vi "IndependentVISApowerDataCollection.vi"() -> ()   [LabVIEW 2019]
uses:
  <vilib>/Utility/file.llb/Write Delimited Spreadsheet (string).vi
  <vilib>/Utility/file.llb/Read Delimited Spreadsheet (string).vi
  <instrlib>/niDigital/niDigital.llb/niDigital Selected Function.ctl
  <instrlib>/niDigital/niDigital.llb/niDigital Output Function.ctl
  Users/Aerolab1/Documents/LabVIEW Data/2019(64-bit)/Projects/TAMU2024/Scripts/KBTR/Independent Digital Control/Bitfield and Data.ctl
  <instrlib>/niDigital/niDigital.llb/niDigital Burst Pattern (Pass Fail).vi
panel:
  in  "BeamEnd":bool
  in  "BeamStart":bool
  out "Register Read (0-64)":u32[](array[numeric])
  out "pass scan":bool[](array[boolean])
  in  "DUT Parameters":T1={"Rx LNA Bias"=4, "Rx Output Amp Bias"=4, "Tx Input PA Bias"=5, "Tx Driver Amp Bias"=1, "Tx Output PA Bias"=5, "Tx, Rx, or OFF?"="Tx", "VGA State"=0, "Swept Together?"=TRUE, "RF Path"="EL0-BM0", "DSA State"=0, "TDU State"=0, "PNA Channel"=1}
  in  "Instrument Handle Out":refnum<k15>
  in  "Reprogram":bool
  in  "Rescan":bool
  in  "KBTR_Collection":bool
  out "RunPath":path
  in  "Run Number":i32
  out "appended array":string[](array[string])
  in  "Head FilePath":path=path "C:/Campaigns/LBNL_Feb_2025/data"
  out "EndRecord":bool
  out "POWER STATUS OUT":bool
  in  "POWER STATUS IN":bool
  out "VISAPowerInfoInputArray":T2(array[cluster])
  out "Status":string
  in  "End Program":bool
  in  "Record Data Toggle":bool
  out "Configuration Echo":string
  out "Parameter Configuration Echo":string[][](array[string])
  in  "Which Channels to Parallelize":u16(ring) items=["I1+I2", "ALL", "I2+I3"]
  in  "Combination Scheme":u16(ring) items=["OFF", "SERIES", "PARALLEL"]
  in  "Voltage Channel 1 (V)":dbl
  in  "Voltage Channel 2 (V)":dbl
  in  "Voltage Channel 3 (V)":dbl
  in  "Current Limit Channel 1 (A)":dbl
  in  "Current Limit Channel 2 (A)":dbl
  in  "Current Limit Channel 3 (A)":dbl
  in  "VISA resource name":refnum<visa-resource-name>
  in  "Apply Power Settings":bool
  # "Run Control and Power Outputs"
  # "Keithley Power Inputs"
  # "Time (H.M.S.####)"
  # "Current (A)"
  # "Voltage (V)"
  # "KBTR configuration (optional)"
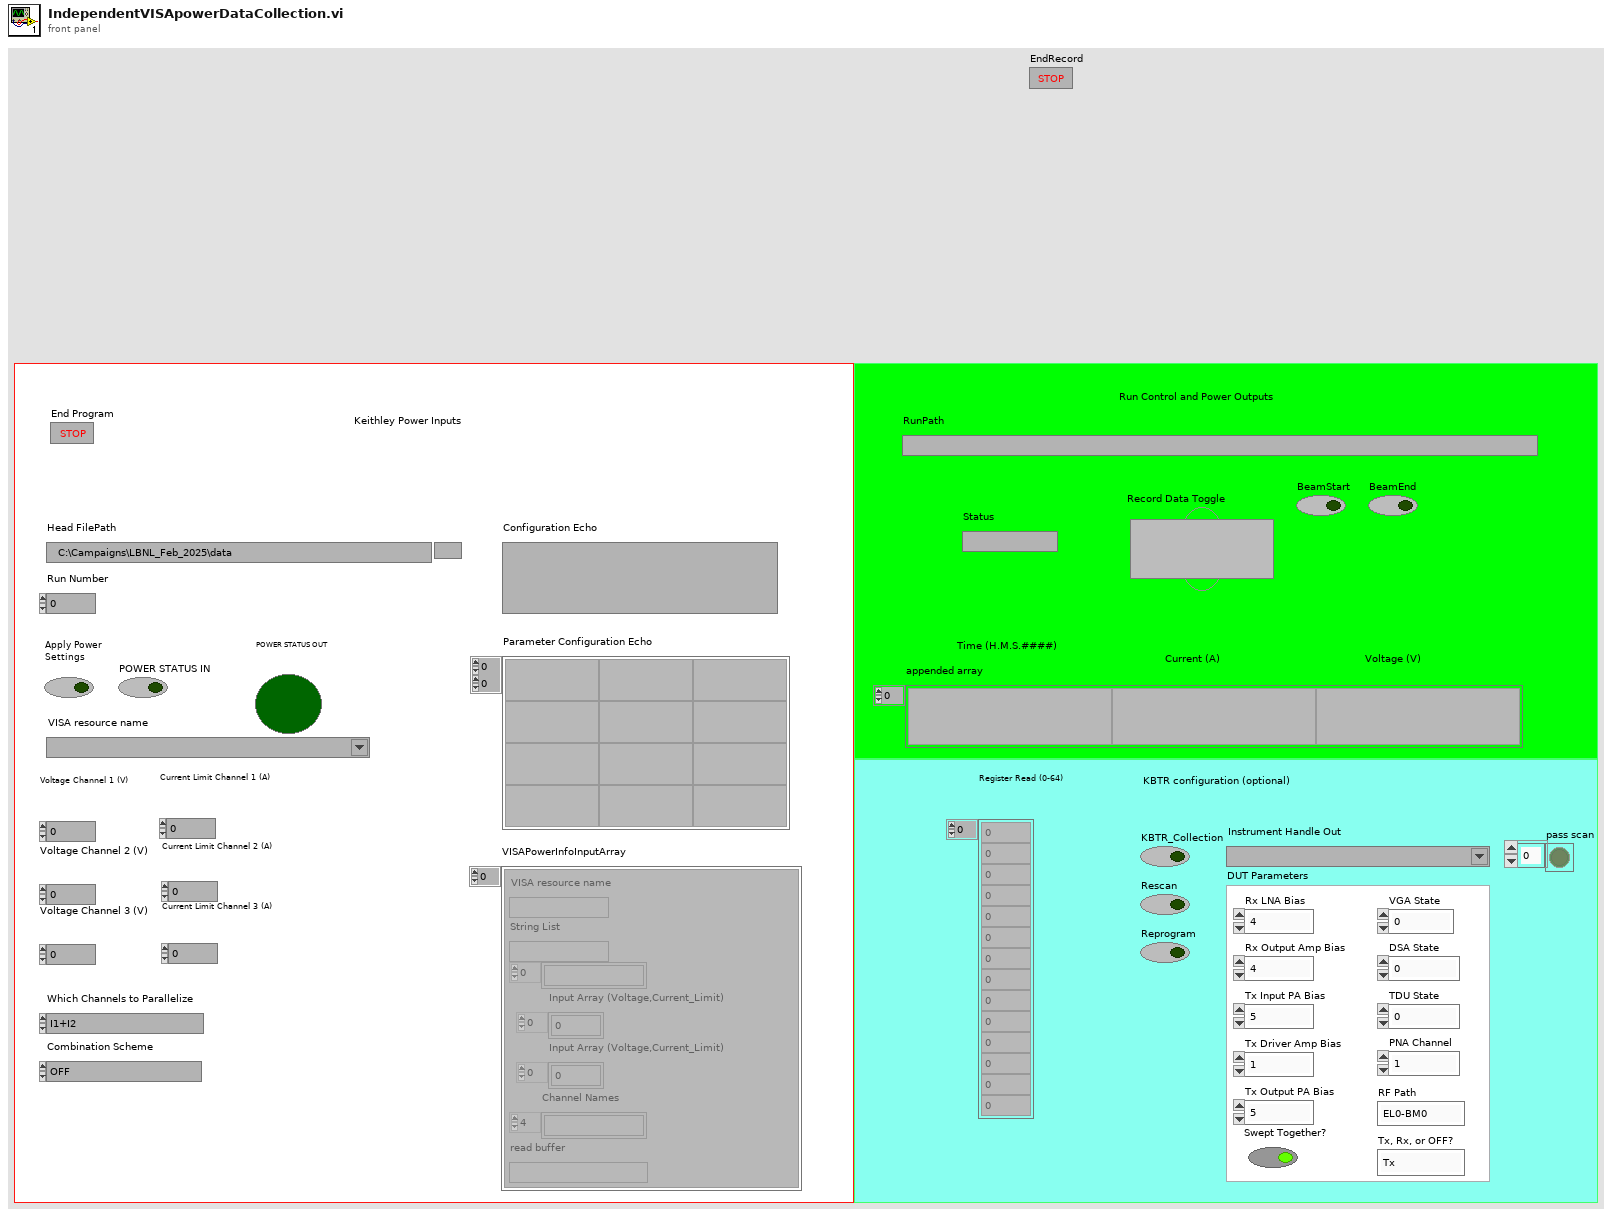
[diagram p1: front panel]
types:
  T1 = cluster{"Rx LNA Bias":i32, "Rx Output Amp Bias":i32, "Tx Input PA Bias":i32, "Tx Driver Amp Bias":i32, "Tx Output PA Bias":i32, "Tx, Rx, or OFF?":string, "VGA State":i32, "Swept Together?":bool, "RF Path":string, "DSA State":i32, "TDU State":i32, "PNA Channel":i32}
  T2 = cluster{"VISA resource name":refnum<visa-resource-name>, "String List":string, string[], "Input Array (Voltage,Current_Limit)":dbl[], "Input Array (Voltage,Current_Limit)":dbl[], "Channel Names":string[], "read buffer":string}[]
  T3 = typedef "Bitfield and Data.ctl" = cluster{"Bitfields":string, "Data":i32}
  T4 = typedef "niDigital Output Function.ctl" = i32
  T5 = typedef "niDigital Selected Function.ctl" = i32
  T6 = enum16{"open", "replace", "create", "open or create", "replace or create", "replace or create with confirmation"}
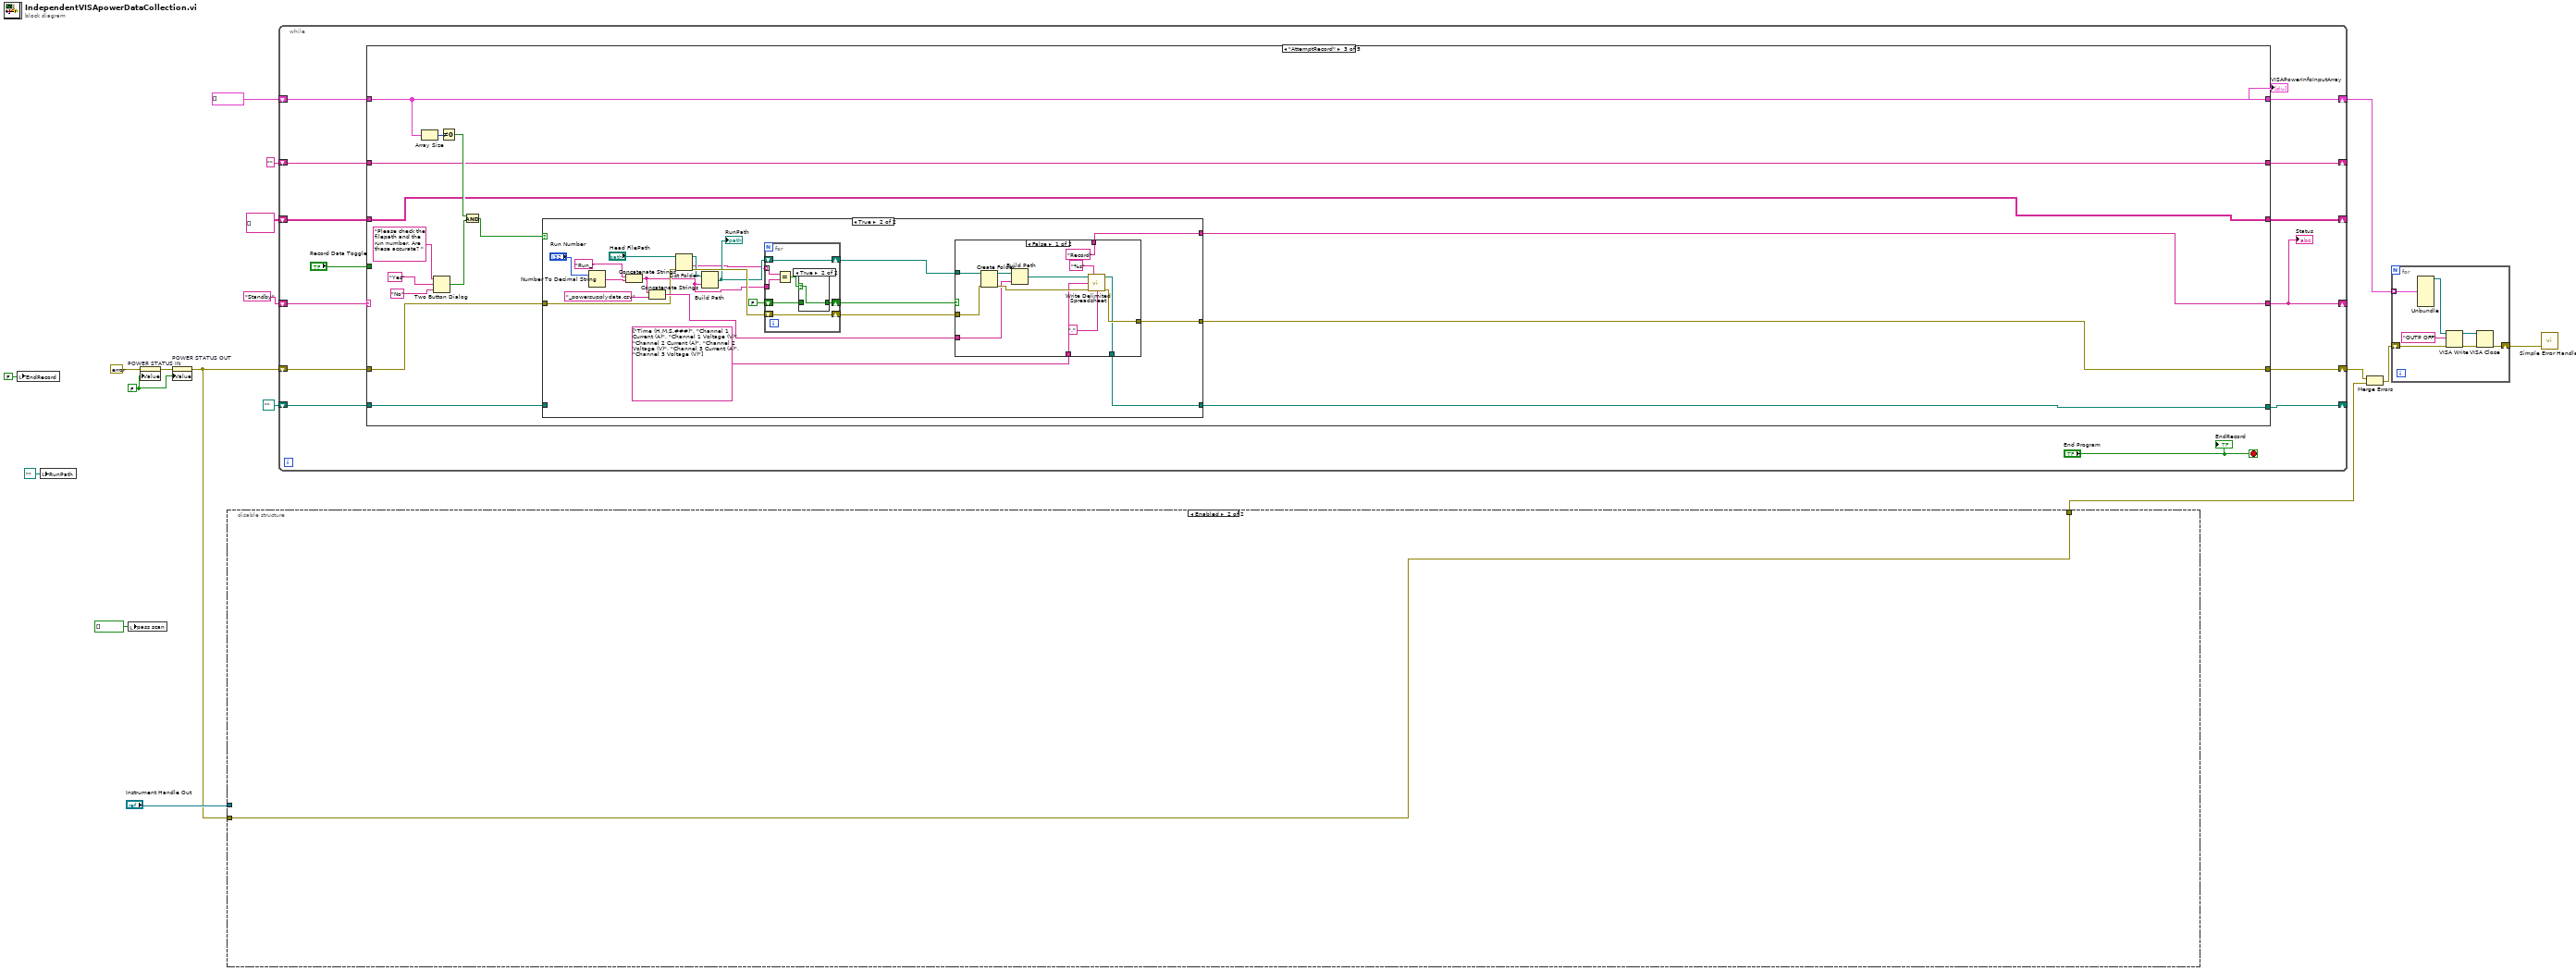
[diagram p0: block diagram]
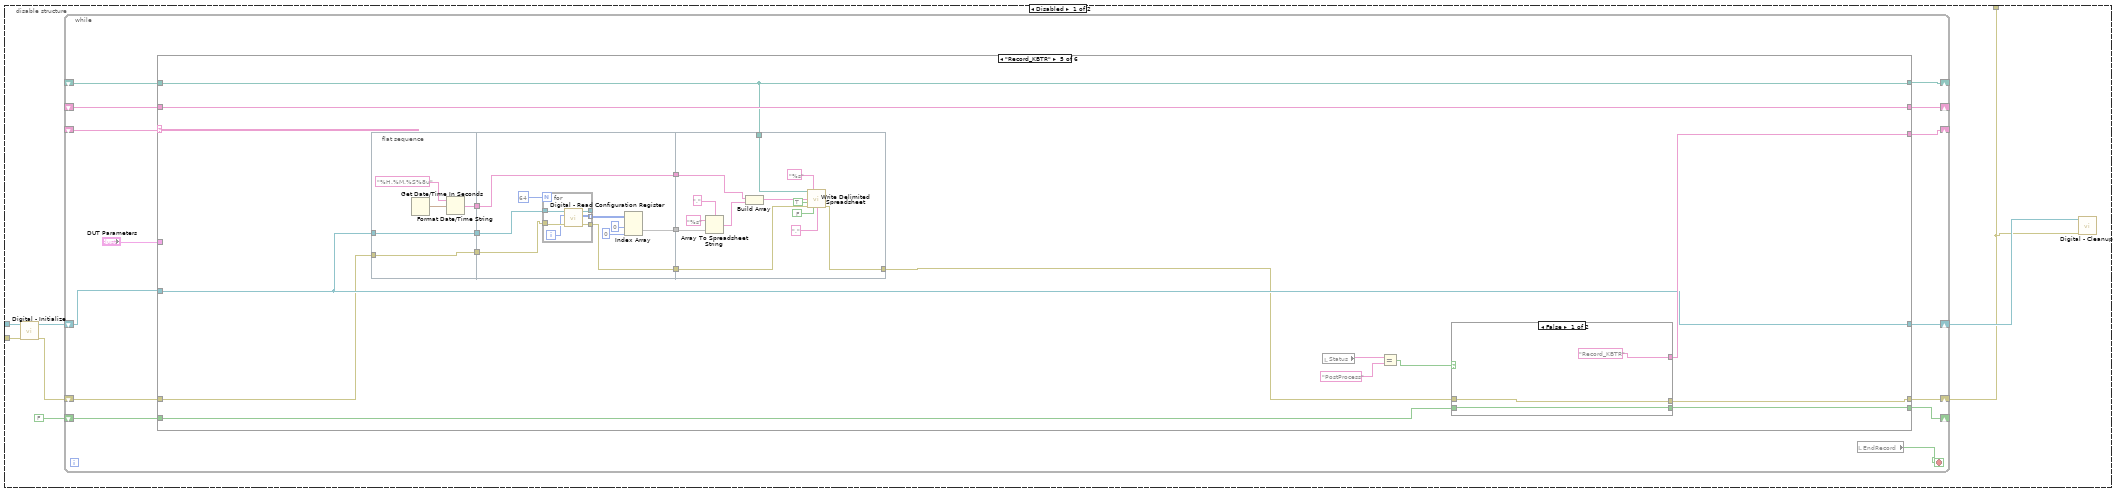
[diagram p2: hidden frame]
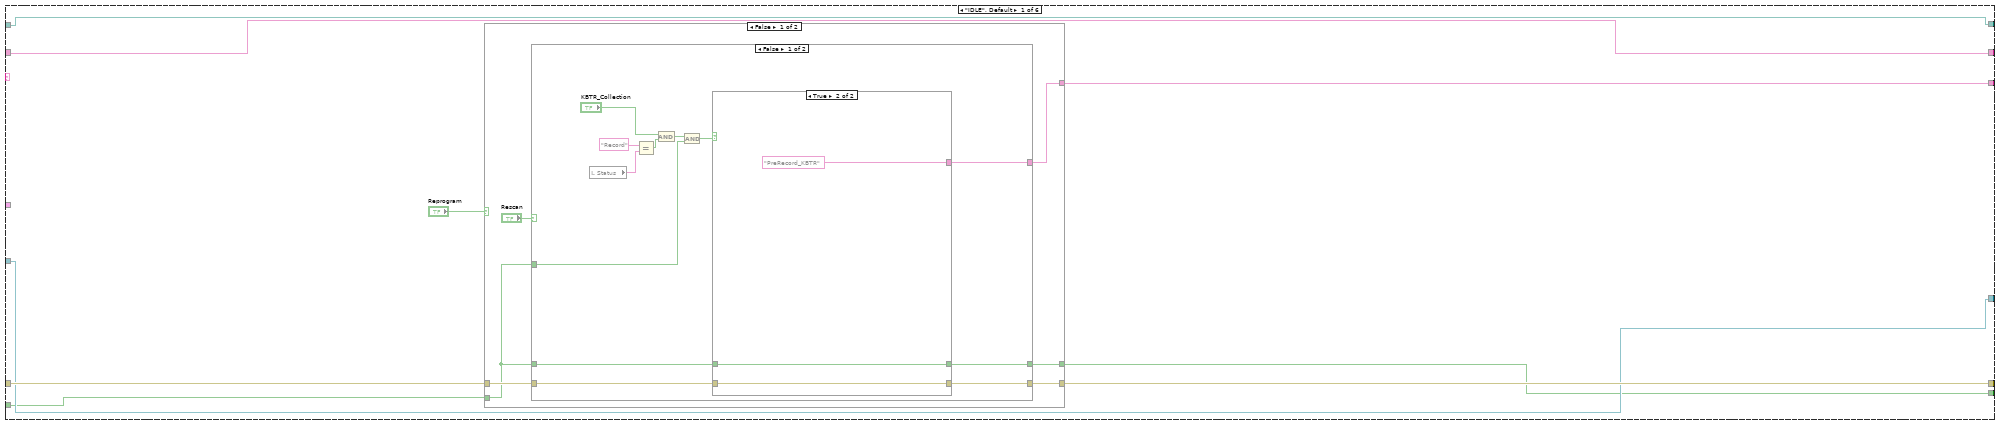
[diagram p3: hidden frame]
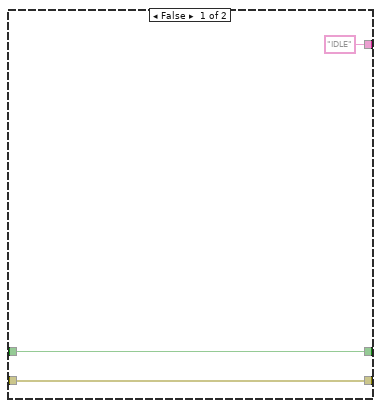
[diagram p4: hidden frame]
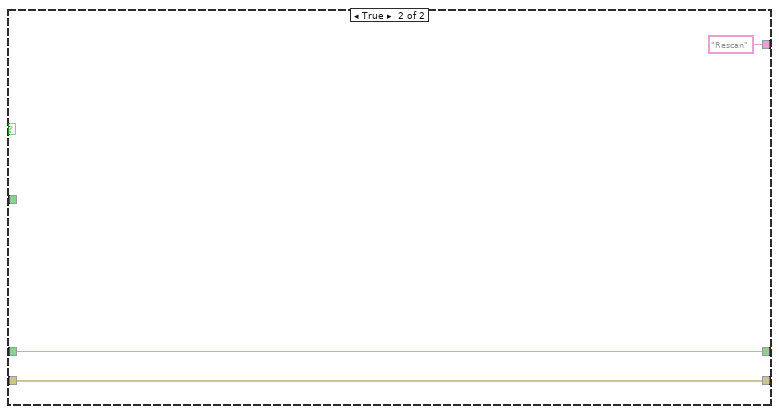
[diagram p5: hidden frame]
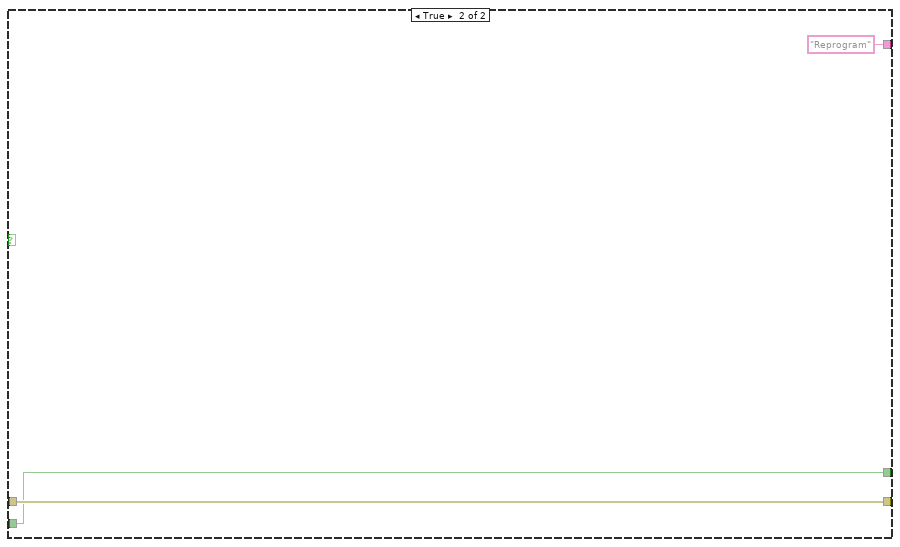
[diagram p6: hidden frame]
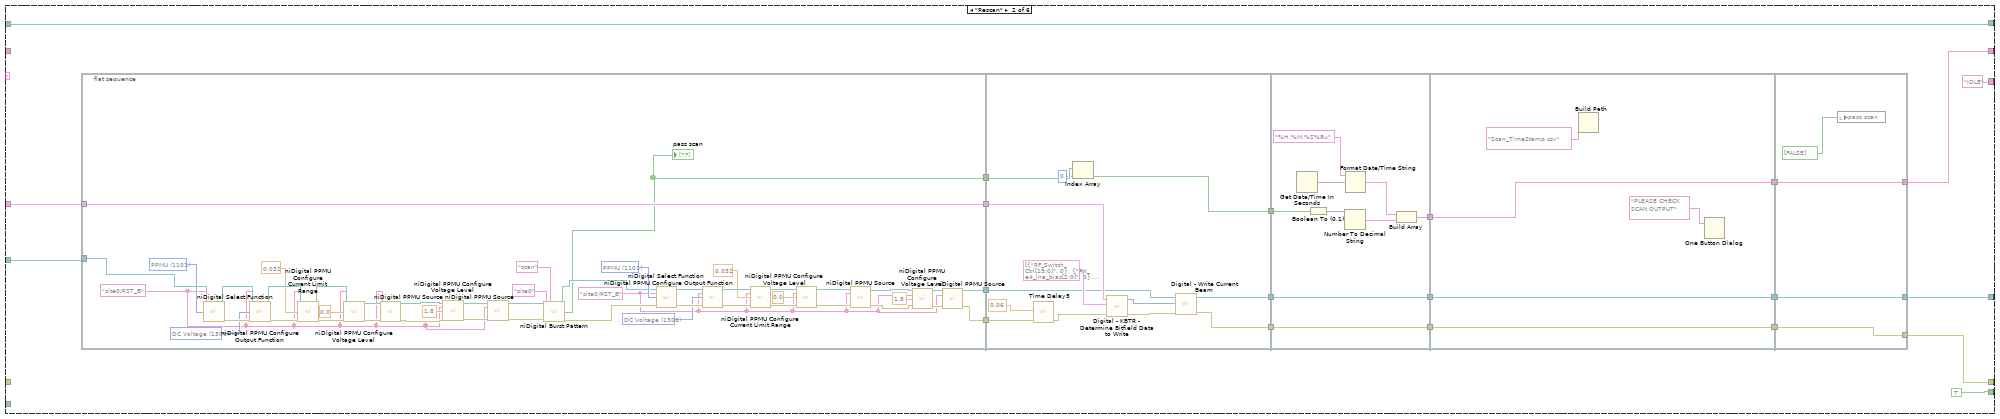
[diagram p7: hidden frame]
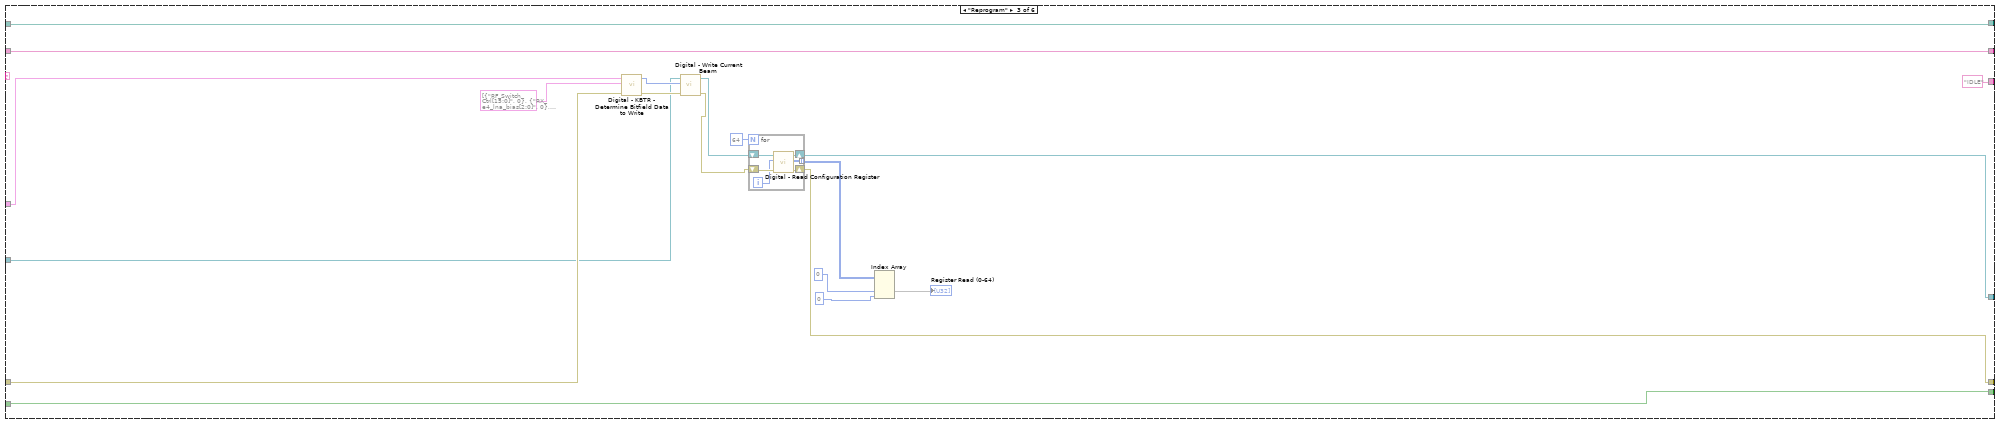
[diagram p8: hidden frame]
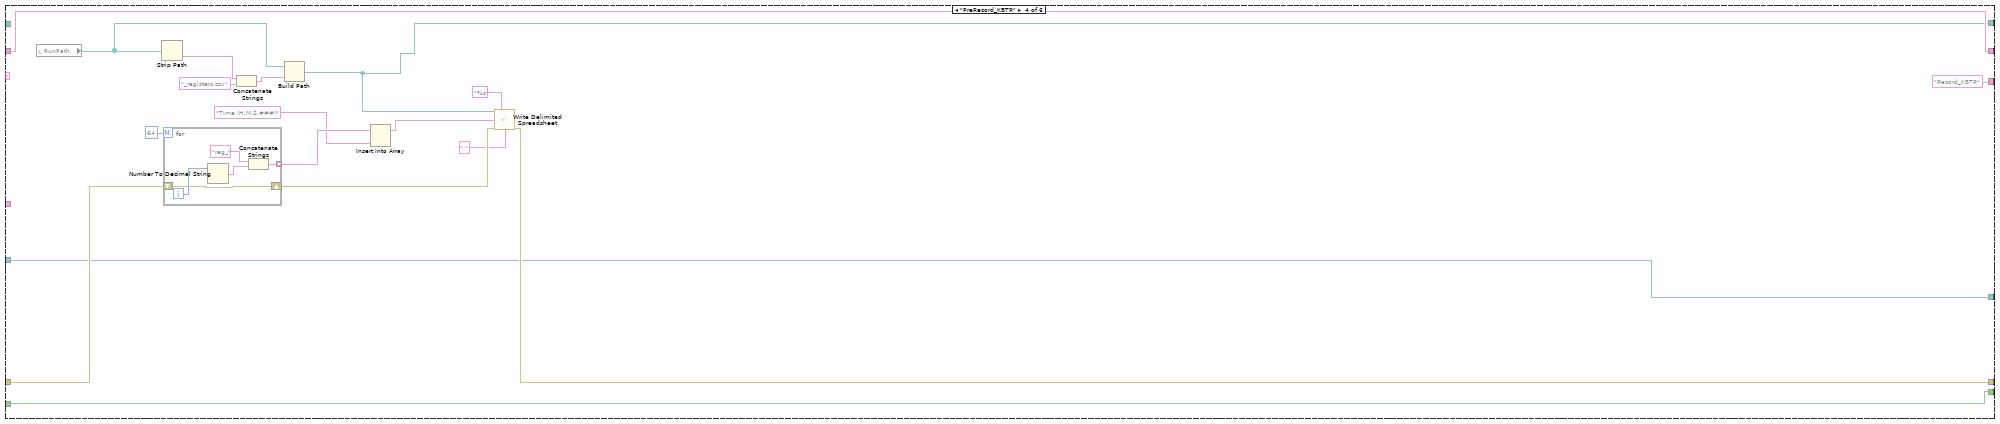
[diagram p9: hidden frame]
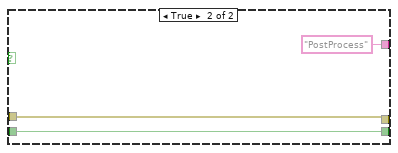
[diagram p10: hidden frame]
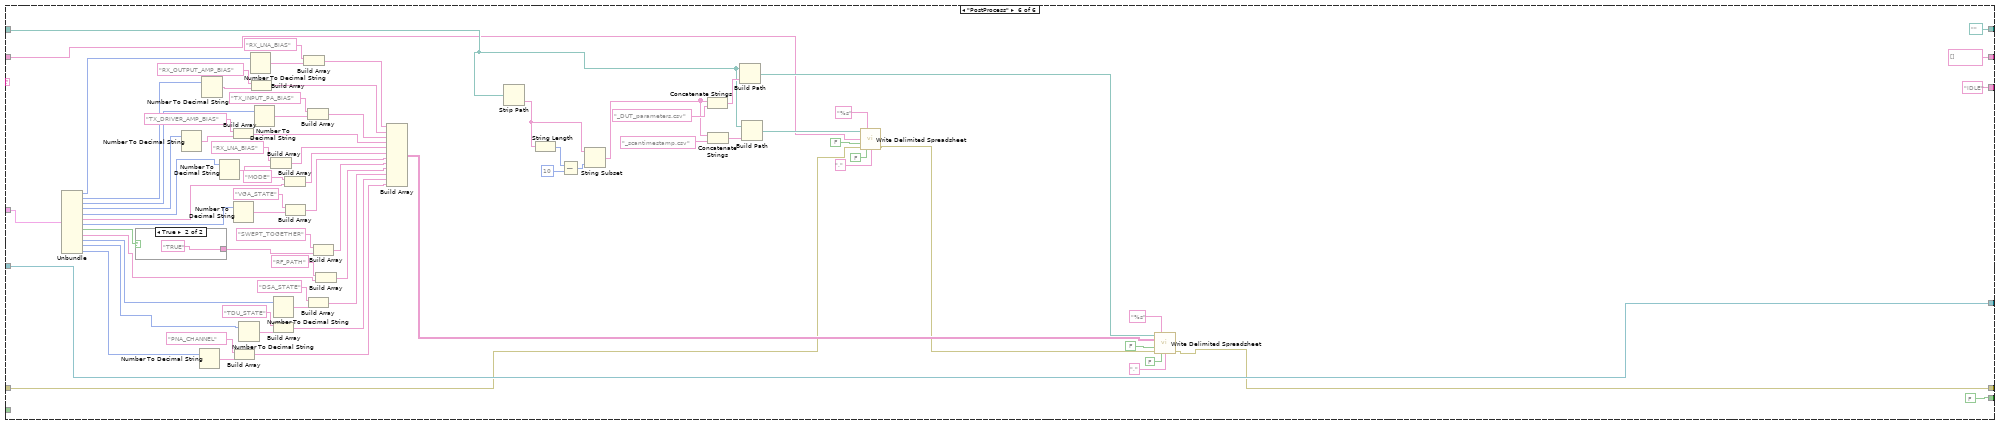
[diagram p11: hidden frame]
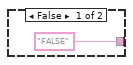
[diagram p12: hidden frame]
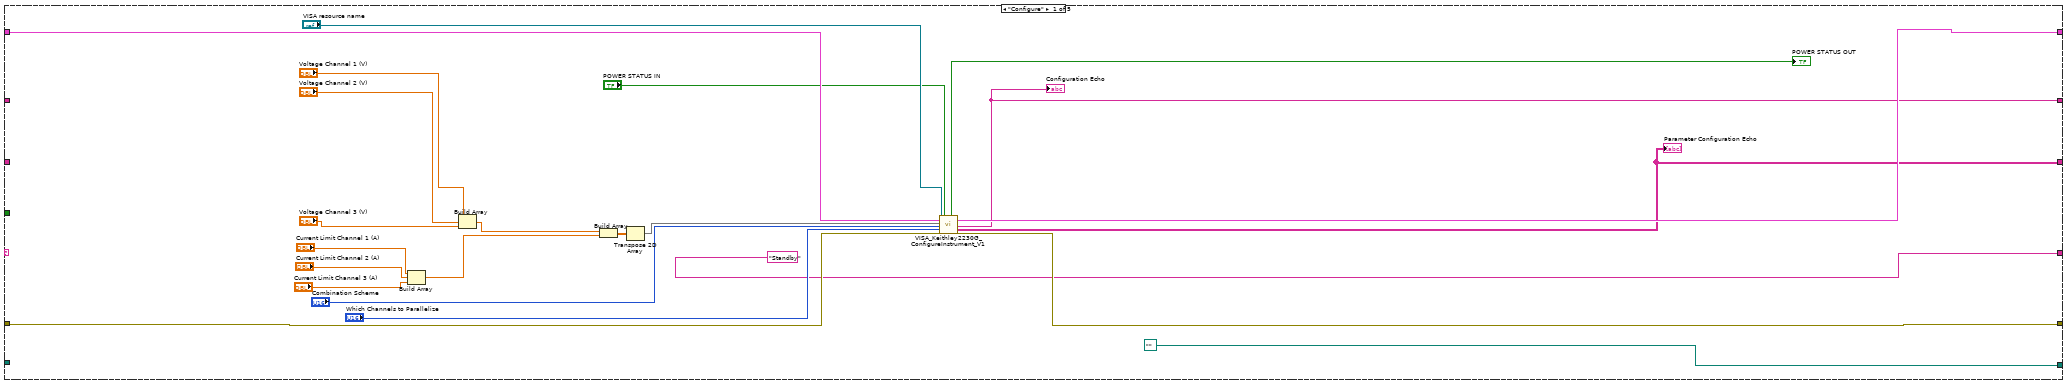
[diagram p13: hidden frame]
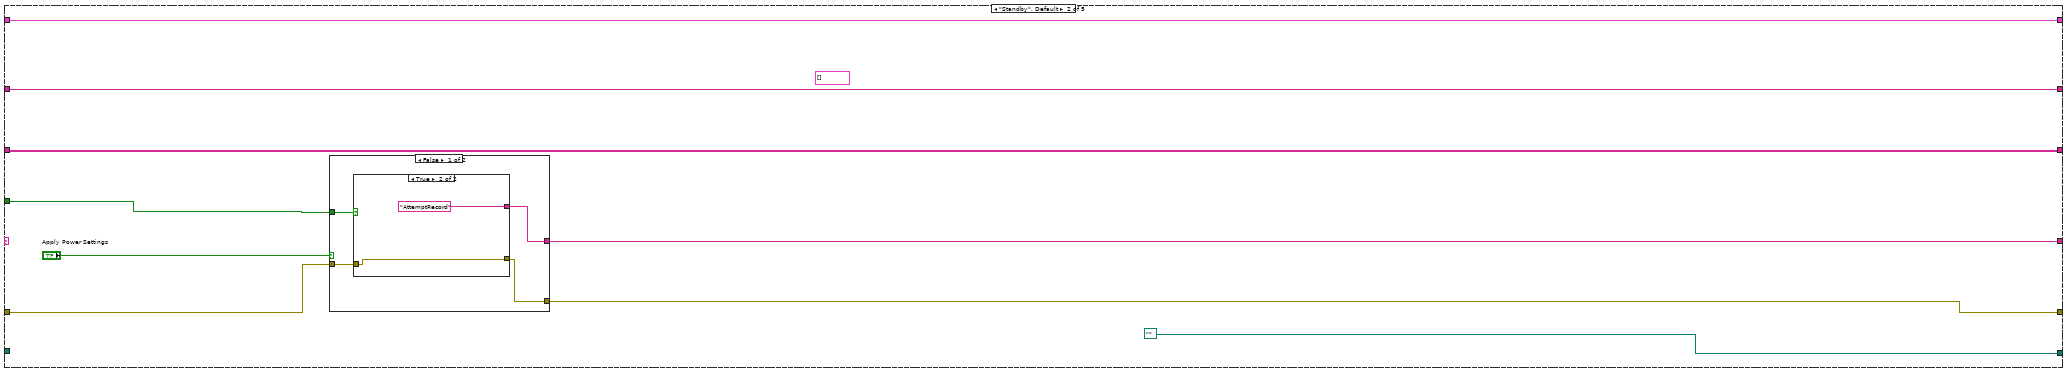
[diagram p14: hidden frame]
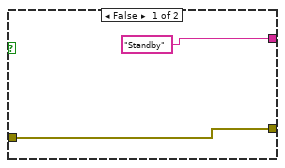
[diagram p15: hidden frame]
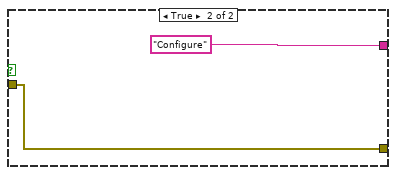
[diagram p16: hidden frame]
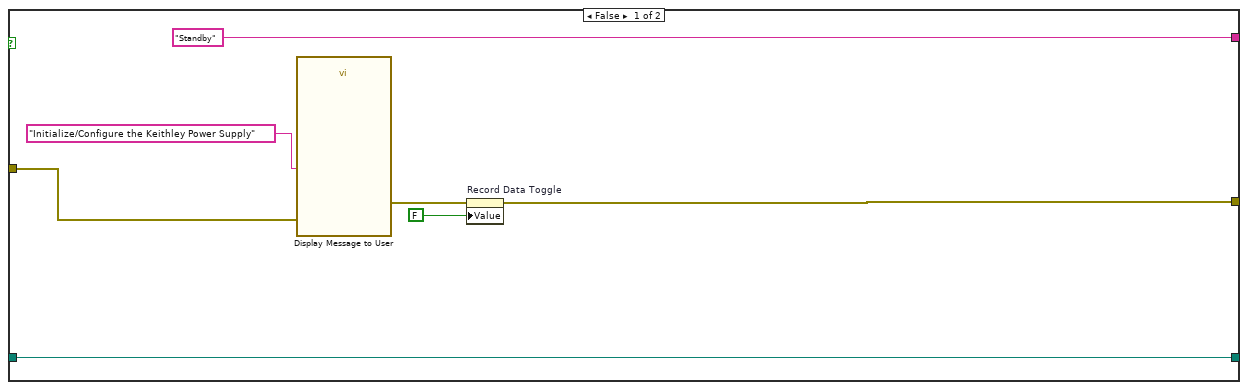
[diagram p17: hidden frame]
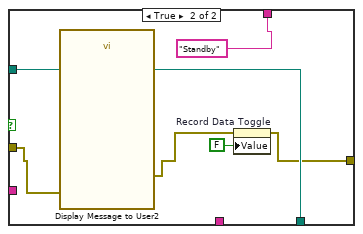
[diagram p18: hidden frame]
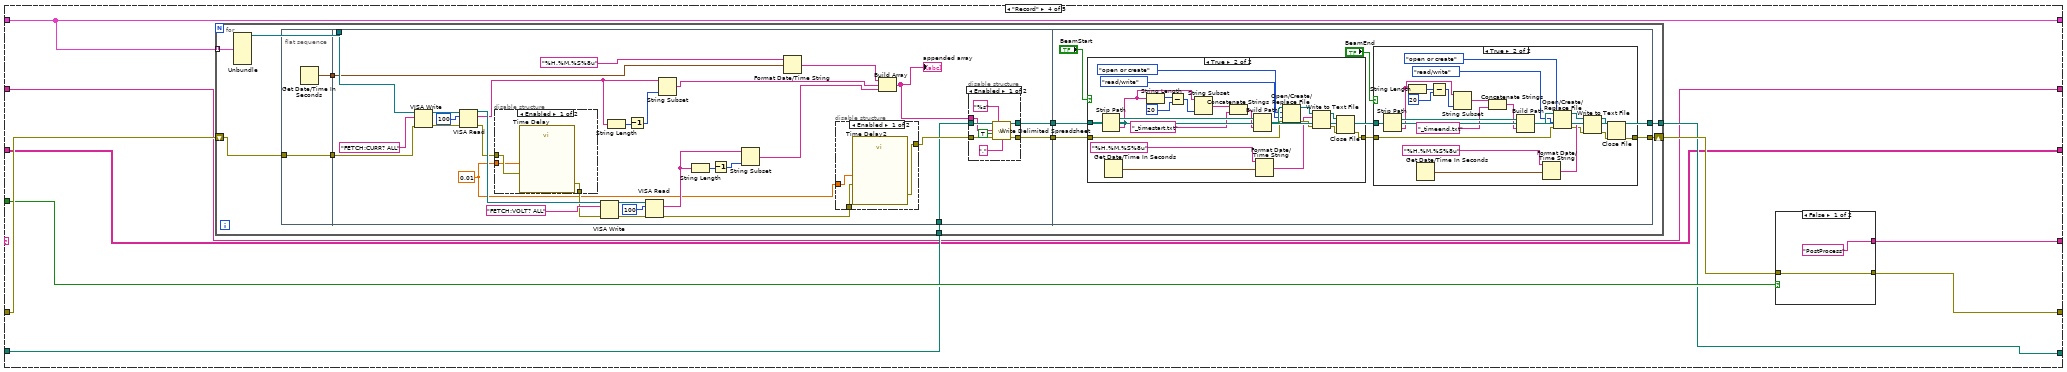
[diagram p20: hidden frame]
diagram:
  w13 = FALSE ("POWER STATUS IN")
  n1 = local write "EndRecord"(FALSE ("EndRecord")) -> ()
  n2 = local write "RunPath"(path "" ("RunPath")) -> ()
  n3 = local write "pass scan"(bool[] [] ("pass scan")) -> ()
  n4 = property on="POWER STATUS IN" class="Bool (strict)"(error in=errorcluster {"status"=FALSE, "code"=0, "source"=""}, "Value"=w13) -> (error out=w14:errorcluster)  [unwired: 1 in, 1 out]
  n5 = property on="POWER STATUS OUT" class="Bool (strict)"(error in=w14, "Value"=w13) -> (error out=w7:errorcluster)  [unwired: 1 in, 1 out]
  n6 = disable-structure shown="Enabled" {
    disable-tunnel: "Instrument Handle Out" -> [w25 _]
    disable-tunnel: w7 -> [w24 w362]
    disable-tunnel: [w19 w362] -> w2
    frame Disabled {
      n7 = call "Digital - Initialize.vi"("Error In"=w24, "Instrument Handle In"=w25) -> ("Error Out"=w23:errorcluster, "Instrument Handle Out"=w21:refnum<k15>)  [unwired: 8 in]
      n8 = while {
        shift-right: [w37] -> _
        shift-left: _ -> [w36]
        shift-right: [w39] -> w19
        shift-left: w23 -> [w38]
        shift-right: [w34] -> w22
        shift-left: w21 -> [w33]
        shift-right: [w31] -> _
        shift-left: FALSE -> [w32]
        shift-right: [w30] -> _
        shift-left: _ -> [w29]
        shift-right: [w28] -> _
        shift-left: _ -> [w27]
        stop <- w26 stop-if-true
        n9 = case shown="\"Record_KBTR\"" w36 {
          tunnel: [w48 w84 w183 w208 w243 w305] -> w39
          tunnel: w38 -> [w47 _ w187 w214 w232 w291]
          tunnel: [w46 "IDLE" "IDLE" "Record_KBTR" w239 "IDLE"] -> w37
          tunnel: w33 -> [w44 w88 w186 w205 w234 w312]
          tunnel: "DUT Parameters" -> [_ w87 w185 _ _ w313]
          tunnel: [w44 w83 w181 w205 w234 w312] -> w34
          tunnel: w32 -> [w43 _ w180 w206 w238 _]
          tunnel: [w42 TRUE w180 w206 w237 FALSE] -> w31
          tunnel: [w41 w79 w179 w204 w227 path "" ("RunPath")] -> w30
          tunnel: w29 -> [w41 w79 w179 _ w227 w297]
          tunnel: [w40 w81 w178 w216 w236 string[] []] -> w28
          tunnel: w27 -> [w40 _ w178 w216 w236 w289]
          frame "IDLE", Default {
            n10 = case shown="False" "Reprogram" {
              tunnel: [w54 w77] -> w48
              tunnel: w47 -> [w53 w77]
              tunnel: [w52 "Reprogram"] -> w46
              tunnel: w43 -> [w49 w76]
              tunnel: [w50 w76] -> w42
              frame False {
                n11 = case shown="False" "Rescan" {
                  tunnel: [w64 w75] -> w54
                  tunnel: w53 -> [w63 w75]
                  tunnel: [w62 "Rescan"] -> w52
                  tunnel: w49 -> [w57 _]
                  tunnel: [w56 w73] -> w50
                  tunnel: w49 -> [w55 w73]
                  frame False {
                    n12 = local read "Status"() -> (w66:string)
                    n13 = Equal?(x="Record", y=w66) -> (x = y?=w61:bool)
                    n14 = And(x="KBTR_Collection", y=w61) -> (x .and. y?=w59:bool)
                    n15 = And(x=w59, y=w57) -> (x .and. y?=w58:bool)
                    n16 = case shown="True" w58 {
                      tunnel: ["IDLE" "PreRecord_KBTR"] -> w62
                      tunnel: [w68 w71] -> w64
                      tunnel: w63 -> [w68 w71]
                      tunnel: [w67 w70] -> w56
                      tunnel: w55 -> [w67 w70]
                      frame False {
                      }
                      frame True {
                      }
                    }
                  }
                  frame True {
                  }
                }
              }
              frame True {
              }
            }
          }
          frame "Rescan" {
            n17 = flat-sequence {
              tunnel: w88 -> [w101]
              tunnel: w87 -> [w146]
              tunnel: [w146] -> w99
              tunnel: [w103] -> w98
              tunnel: [w102] -> w97
              tunnel: [w100] -> w96
              tunnel: w99 -> [w156]
              tunnel: w98 -> [w155]
              tunnel: w97 -> [w151]
              tunnel: [w147] -> w95
              tunnel: w96 -> [w154]
              tunnel: [w152] -> w94
              tunnel: [w148] -> w93
              tunnel: w95 -> [w168]
              tunnel: [w168] -> w92
              tunnel: w94 -> [w166]
              tunnel: [w161] -> w91
              tunnel: [w160] -> w90
              tunnel: w93 -> [w160]
              tunnel: [w172] -> w89
              tunnel: [w171] -> w85
              tunnel: [w170] -> w80
              tunnel: w90 -> [w171]
              tunnel: w91 -> [w170]
              tunnel: w92 -> [w172]
              tunnel: [w177] -> w83
              tunnel: w89 -> [w177]
              tunnel: [w175] -> w84
              tunnel: w85 -> [w175]
              tunnel: [w174] -> w81
              tunnel: w80 -> [w174]
              frame #0 {
                w124 = T4 1300 items=["DC Voltage"=1300, "DC Current"=1301] ("output function")
                w104 = "site0/RST_B" ("channel list")
                w133 = T5 1101 items=["Digital"=1100, "PPMU"=1101, "Off"=1102, "Disconnect"=1103] ("function")
                w134 = T4 1300 items=["DC Voltage"=1300, "DC Current"=1301] ("output function")
                w112 = "site0/RST_B" ("channel list")
                w143 = T5 1101 items=["Digital"=1100, "PPMU"=1101, "Off"=1102, "Disconnect"=1103] ("function")
                n18 = call <instrlib>:"niDigital Select Function.vi"("instrument handle"=w101, "channel list"=w112, "function"=w143) -> ("instrument handle out"=w142:refnum<k15>, "error out"=w137:errorcluster)  [unwired: 11 in]
                n19 = call <instrlib>:"niDigital PPMU Configure Output Function.vi"("instrument handle"=w142, "channel list"=w112, "output function"=w134, "error in"=w137) -> ("instrument handle out"=w141:refnum<k15>, "error out"=w138:errorcluster)  [unwired: 10 in]
                n20 = call <instrlib>:"niDigital PPMU Configure Current Limit Range.vi"("instrument handle"=w141, "channel list"=w112, "current limit range (A)"=0.032 ("current limit (A)"), "error in"=w138) -> ("instrument handle out"=w140:refnum<k15>, "error out"=w139:errorcluster)  [unwired: 10 in]
                n21 = call <instrlib>:"niDigital PPMU Configure Voltage Level.vi"("instrument handle"=w140, "channel list"=w112, "voltage level (V)"=0.0, "error in"=w139) -> ("instrument handle out"=w118:refnum<k15>, "error out"=w117:errorcluster)  [unwired: 10 in]
                n22 = call <instrlib>:"niDigital PPMU Source.vi"("instrument handle"=w118, "channel list"=w112, "error in"=w117) -> ("instrument handle out"=w116:refnum<k15>, "error out"=w115:errorcluster)  [unwired: 11 in]
                n23 = call <instrlib>:"niDigital PPMU Configure Voltage Level.vi"("instrument handle"=w116, "channel list"=w112, "voltage level (V)"=1.8, "error in"=w115) -> ("instrument handle out"=w113:refnum<k15>, "error out"=w114:errorcluster)  [unwired: 10 in]
                n24 = call <instrlib>:"niDigital PPMU Source.vi"("instrument handle"=w113, "channel list"=w112, "error in"=w114) -> ("instrument handle out"=w110:refnum<k15>, "error out"=w111:errorcluster)  [unwired: 11 in]
                n25 = call-poly <instrlib>:"niDigital Burst Pattern.vi"("instrument handle"=w110, "start label"="scan", "site list"="site0", "error in"=w111) -> ("instrument handle out"=w120:refnum<k15>, "pass"=w100:bool[], "error out"=w121:errorcluster)  [unwired: 9 in]
                "pass scan" <- w100
                n26 = call <instrlib>:"niDigital Select Function.vi"("instrument handle"=w120, "channel list"=w104, "function"=w133, "error in"=w121) -> ("instrument handle out"=w132:refnum<k15>, "error out"=w127:errorcluster)  [unwired: 10 in]
                n27 = call <instrlib>:"niDigital PPMU Configure Output Function.vi"("instrument handle"=w132, "channel list"=w104, "output function"=w124, "error in"=w127) -> ("instrument handle out"=w131:refnum<k15>, "error out"=w128:errorcluster)  [unwired: 10 in]
                n28 = call <instrlib>:"niDigital PPMU Configure Current Limit Range.vi"("instrument handle"=w131, "channel list"=w104, "current limit range (A)"=0.032 ("current limit (A)"), "error in"=w128) -> ("instrument handle out"=w130:refnum<k15>, "error out"=w129:errorcluster)  [unwired: 10 in]
                n29 = call <instrlib>:"niDigital PPMU Configure Voltage Level.vi"("instrument handle"=w130, "channel list"=w104, "voltage level (V)"=0.0, "error in"=w129) -> ("instrument handle out"=w122:refnum<k15>, "error out"=w123:errorcluster)  [unwired: 10 in]
                n30 = call <instrlib>:"niDigital PPMU Source.vi"("instrument handle"=w122, "channel list"=w104, "error in"=w123) -> ("instrument handle out"=w105:refnum<k15>, "error out"=w106:errorcluster)  [unwired: 11 in]
                n31 = call <instrlib>:"niDigital PPMU Configure Voltage Level.vi"("instrument handle"=w105, "channel list"=w104, "voltage level (V)"=1.8, "error in"=w106) -> ("instrument handle out"=w109:refnum<k15>, "error out"=w108:errorcluster)  [unwired: 10 in]
                n32 = call <instrlib>:"niDigital PPMU Source.vi"("instrument handle"=w109, "channel list"=w104, "error in"=w108) -> ("instrument handle out"=w102:refnum<k15>, "error out"=w103:errorcluster)  [unwired: 11 in]
              }
              frame #1 {
                n33 = call "Time Delay5"("error in (no error)"=w155, "Delay Time (s)"=0.06) -> ("error out"=w159:errorcluster)  [unwired: 9 in]
                n34 = Index Array(array=w154, index=0) -> (element=w152:bool)
                n35 = call "Digital - KBTR - Determine Bitfield Data to Write.vi"("Error In"=w159, "Initial Data"=T3[] [{"Bitfields"="RF_Switch_Ctrl[15:0]", "Data"=0}, {"Bitfields"="RX_e4_lna_bias[2:0]", "Data"=0}, {"Bitfields"="RX_e3_lna_bias[2:0]", "Data"=0}, {"Bitfields"="RX_e2_lna_bias[2:0]", "Data"=0}, {"Bitfields"="RX_e1_lna_bias[2:0]", "Data"=0}, {"Bitfields"="RX_b1_gb_bias[2:0]", "Data"=0}, {"Bitfields"="TX_e4_gb_bias[2:0]", "Data"=0}, {"Bitfields"="TX_e3_gb_bias[2:0]", "Data"=0}, {"Bitfields"="TX_e2_gb_bias[2:0]", "Data"=0}, {"Bitfields"="TX_e1_gb_bias[2:0]", "Data"=0}, {"Bitfields"="TX_e4_pa_bias[2:0]", "Data"=0}, {"Bitfields"="TX_e3_pa_bias[2:0]", "Data"=0}, {"Bitfields"="TX_e2_pa_bias[2:0]", "Data"=0}, {"Bitfields"="TX_e1_pa_bias[2:0]", "Data"=0}, {"Bitfields"="TX_b1_pa_bias[2:0]", "Data"=0}, {"Bitfields"="TX_e4_gb_attn[3:0]", "Data"=0}, {"Bitfields"="TX_e3_gb_attn[3:0]", "Data"=0}, {"Bitfields"="TX_e2_gb_attn[3:0]", "Data"=0}, {"Bitfields"="TX_e1_gb_attn[3:0]", "Data"=0}, {"Bitfields"="RX_e4_lna_en", "Data"=0}, {"Bitfields"="RX_e3_lna_en", "Data"=0}, {"Bitfields"="RX_e2_lna_en", "Data"=0}, {"Bitfields"="RX_e1_lna_en", "Data"=0}, {"Bitfields"="RX_b1_gb_en", "Data"=0}, {"Bitfields"="TX_e4_gb_en", "Data"=0}, {"Bitfields"="TX_e3_gb_en", "Data"=0}, {"Bitfields"="TX_e2_gb_en", "Data"=0}, {"Bitfields"="TX_e1_gb_en", "Data"=0}, {"Bitfields"="TX_e4_pa_en", "Data"=0}, {"Bitfields"="TX_e3_pa_en", "Data"=0}, {"Bitfields"="TX_e2_pa_en", "Data"=0}, {"Bitfields"="TX_e1_pa_en", "Data"=0}, {"Bitfields"="TX_b1_pa_en", "Data"=0}, {"Bitfields"="Time_D[5:0]", "Data"=0}, {"Bitfields"="Time_C[5:0]", "Data"=0}, {"Bitfields"="Time_B[5:0]", "Data"=0}, {"Bitfields"="Time_A[5:0]", "Data"=0}, {"Bitfields"="Attn_D[5:0]", "Data"=0}, {"Bitfields"="Attn_C[5:0]", "Data"=0}, {"Bitfields"="Attn_B[5:0]", "Data"=0}, {"Bitfields"="Attn_A[5:0]", "Data"=0}], "DUT Parameters"=w156) -> ("Error Out"=w149:errorcluster, "Data Stream Out"=w150:u32[])  [unwired: 7 in]
                n36 = call "Digital - Write Current Beam.vi"("Error In"=w149, "Data In"=w150, "Instrument Handle In"=w151) -> ("Error Out"=w148:errorcluster, "Instrument Handle Out"=w147:refnum<k15>)  [unwired: 7 in]
              }
              frame #2 {
                n37 = Get Date/Time In Seconds() -> (seconds since 1Jan1904=w167:timestamp)
                n38 = Boolean To (0,1)(Boolean=w166) -> (0, 1=w165:i16)
                n39 = Number To Decimal String(number=w165) -> (decimal integer string=w163:string)  [unwired: 1 in]
                n40 = Format Date/Time String(time format string (%c)="%H.%M.%S%8u", seconds (now)=w167) -> (date/time string=w162:string)  [unwired: 1 in]
                n41 = Build Array(w162, w163) -> (w161:string[])
              }
              frame #3 {
                n42 = Build Path(name or relative path="Scan_TimeStamp.csv") -> ()  [unwired: 1 in, 1 out]
                n43 = One Button Dialog(message="PLEASE CHECK SCAN OUTPUT") -> ()  [unwired: 1 in, 1 out]
              }
              frame #4 {
                n44 = local write "pass scan"(bool[] [FALSE] ("PASS_SCAN")) -> ()
              }
            }
          }
          frame "Reprogram" {
            n45 = call "Digital - KBTR - Determine Bitfield Data to Write.vi"("Error In"=w187, "Initial Data"=T3[] [{"Bitfields"="RF_Switch_Ctrl[15:0]", "Data"=0}, {"Bitfields"="RX_e4_lna_bias[2:0]", "Data"=0}, {"Bitfields"="RX_e3_lna_bias[2:0]", "Data"=0}, {"Bitfields"="RX_e2_lna_bias[2:0]", "Data"=0}, {"Bitfields"="RX_e1_lna_bias[2:0]", "Data"=0}, {"Bitfields"="RX_b1_gb_bias[2:0]", "Data"=0}, {"Bitfields"="TX_e4_gb_bias[2:0]", "Data"=0}, {"Bitfields"="TX_e3_gb_bias[2:0]", "Data"=0}, {"Bitfields"="TX_e2_gb_bias[2:0]", "Data"=0}, {"Bitfields"="TX_e1_gb_bias[2:0]", "Data"=0}, {"Bitfields"="TX_e4_pa_bias[2:0]", "Data"=0}, {"Bitfields"="TX_e3_pa_bias[2:0]", "Data"=0}, {"Bitfields"="TX_e2_pa_bias[2:0]", "Data"=0}, {"Bitfields"="TX_e1_pa_bias[2:0]", "Data"=0}, {"Bitfields"="TX_b1_pa_bias[2:0]", "Data"=0}, {"Bitfields"="TX_e4_gb_attn[3:0]", "Data"=0}, {"Bitfields"="TX_e3_gb_attn[3:0]", "Data"=0}, {"Bitfields"="TX_e2_gb_attn[3:0]", "Data"=0}, {"Bitfields"="TX_e1_gb_attn[3:0]", "Data"=0}, {"Bitfields"="RX_e4_lna_en", "Data"=0}, {"Bitfields"="RX_e3_lna_en", "Data"=0}, {"Bitfields"="RX_e2_lna_en", "Data"=0}, {"Bitfields"="RX_e1_lna_en", "Data"=0}, {"Bitfields"="RX_b1_gb_en", "Data"=0}, {"Bitfields"="TX_e4_gb_en", "Data"=0}, {"Bitfields"="TX_e3_gb_en", "Data"=0}, {"Bitfields"="TX_e2_gb_en", "Data"=0}, {"Bitfields"="TX_e1_gb_en", "Data"=0}, {"Bitfields"="TX_e4_pa_en", "Data"=0}, {"Bitfields"="TX_e3_pa_en", "Data"=0}, {"Bitfields"="TX_e2_pa_en", "Data"=0}, {"Bitfields"="TX_e1_pa_en", "Data"=0}, {"Bitfields"="TX_b1_pa_en", "Data"=0}, {"Bitfields"="Time_D[5:0]", "Data"=0}, {"Bitfields"="Time_C[5:0]", "Data"=0}, {"Bitfields"="Time_B[5:0]", "Data"=0}, {"Bitfields"="Time_A[5:0]", "Data"=0}, {"Bitfields"="Attn_D[5:0]", "Data"=0}, {"Bitfields"="Attn_C[5:0]", "Data"=0}, {"Bitfields"="Attn_B[5:0]", "Data"=0}, {"Bitfields"="Attn_A[5:0]", "Data"=0}], "DUT Parameters"=w185) -> ("Error Out"=w188:errorcluster, "Data Stream Out"=w191:u32[])  [unwired: 7 in]
            n46 = call "Digital - Write Current Beam.vi"("Error In"=w188, "Data In"=w191, "Instrument Handle In"=w186) -> ("Error Out"=w189:errorcluster, "Instrument Handle Out"=w190:refnum<k15>)  [unwired: 7 in]
            n47 = for {
              N: 64 -> [_]
              tunnel: [w199] -> w195 mode=indexing
              shift-right: [w201] -> w181
              shift-left: w190 -> [w202]
              shift-right: [w200] -> w183
              shift-left: w189 -> [w198]
              i -> [w197]
              n48 = call "Digital - Read Configuration Register.vi"("Error In"=w198, "Register Address"=w197, "Instrument Handle In"=w202) -> ("Error Out"=w200:errorcluster, "Data Out"=w199:u32[][], "Instrument Handle Out"=w201:refnum<k15>)  [unwired: 6 in]
            }
            n49 = Index Array(array=w195, index (dim 1)=0 ("index (col)"), index (dim 2)=0 ("disabled index (col)")) -> (element=→"Register Read (0-64)":u32[])  [unwired: 1 in]
          }
          frame "PreRecord_KBTR" {
            n50 = local read "RunPath"() -> (w215:path)
            n51 = Strip Path(path=w215) -> (name=w219:string)  [unwired: 1 out]
            n52 = for {
              N: 64 -> [_]
              shift-right: [w224] -> w213
              shift-left: w214 -> [w224]
              tunnel: [w221] -> w212 mode=indexing
              i -> [w225]
              n53 = Number To Decimal String(number=w225) -> (decimal integer string=w223:string)  [unwired: 1 in]
              n54 = Concatenate Strings("reg_" ("string"), w223) -> (w221:string)
            }
            n55 = Concatenate Strings(w219, "_registers.csv" ("string")) -> (w217:string)
            n56 = Build Path(base path=w215, name or relative path=w217) -> (appended path=w204:path)
            n57 = Insert Into Array(array=w212, new element="Time (H.M.S.###)" ("new element/subarray")) -> (w210:string[])  [unwired: 1 in]
            n58 = call-poly <vilib>:"Write Delimited Spreadsheet.vi"("file path (dialog if empty)"=w204, "format (%s)"="%s", "1D data"=w210, "error in (no error)"=w213, "delimiter (\\t)"="," ("delimiter (\\t)")) -> ("error out"=w208:errorcluster)  [unwired: 9 in, 1 out]
          }
          frame "Record_KBTR" {
            n59 = flat-sequence {
              tunnel: [w246] -> w235
              tunnel: w234 -> [w246]
              tunnel: [w245] -> w233
              tunnel: w232 -> [w245]
              tunnel: [w244] -> w228
              tunnel: w235 -> [w253]
              tunnel: w233 -> [w252]
              tunnel: [w251] -> w231
              tunnel: [w250] -> w230
              tunnel: [w249] -> w229
              tunnel: w228 -> [w249]
              tunnel: [w265] -> w226
              tunnel: w231 -> [w268]
              tunnel: w230 -> [w274]
              tunnel: w229 -> [w272]
              tunnel: w227 -> [w264]
              frame #0 {
                n60 = Get Date/Time In Seconds() -> (seconds since 1Jan1904=w248:timestamp)
                n61 = Format Date/Time String(time format string (%c)="%H.%M.%S%8u", seconds (now)=w248) -> (date/time string=w244:string)  [unwired: 1 in]
              }
              frame #1 {
                n62 = for {
                  N: 64 -> [_]
                  tunnel: w253 -> [w263]
                  tunnel: [w262] -> _
                  tunnel: [w261] -> w251
                  tunnel: [w260] -> w257 mode=indexing
                  tunnel: w252 -> [w259]
                  i -> [w258]
                  n63 = call "Digital - Read Configuration Register.vi"("Error In"=w259, "Register Address"=w258, "Instrument Handle In"=w263) -> ("Error Out"=w261:errorcluster, "Data Out"=w260:u32[][], "Instrument Handle Out"=w262:refnum<k15>)  [unwired: 6 in]
                }
                n64 = Index Array(array=w257, index (dim 1)=0 ("index (col)"), index (dim 2)=0 ("disabled index (col)")) -> (element=w250:u32[])  [unwired: 1 in]
              }
              frame #2 {
                n65 = Array To Spreadsheet String(delimiter (Tab)=",", array=w274, 3:"%s" ("format string")) -> (spreadsheet string=w273:string)
                n66 = Build Array(w272, w273) -> (w271:string[])
                n67 = call-poly <vilib>:"Write Delimited Spreadsheet.vi"("file path (dialog if empty)"=w264, "format (%s)"="%s", "1D data"=w271, "append to file? (new file:F)"=TRUE, "error in (no error)"=w268, "transpose? (no:F)"=FALSE, "delimiter (\\t)"="," ("delimiter (\\t)")) -> ("error out"=w265:errorcluster)  [unwired: 7 in, 1 out]
              }
            }
            n68 = local read "Status"() -> (w242:string)
            n69 = Equal?(x=w242, y="PostProcess") -> (x = y?=w240:bool)
            n70 = case shown="False" w240 {
              tunnel: [w279 w282] -> w243
              tunnel: w226 -> [w279 w282]
              tunnel: ["Record_KBTR" "PostProcess"] -> w239
              tunnel: w238 -> [w277 w280]
              tunnel: [w277 w280] -> w237
              frame False {
              }
              frame True {
              }
            }
          }
          frame "PostProcess" {
            n71 = Unbundle(w313) -> ("Rx LNA Bias"=w359:i32, "Rx Output Amp Bias"=w354:i32, "Tx Input PA Bias"=w351:i32, "Tx Driver Amp Bias"=w348:i32, "Tx Output PA Bias"=w347:i32, "Tx, Rx, or OFF?"=w343:string, "VGA State"=w342:i32, "Swept Together?"=w338:bool, "RF Path"=w335:string, "DSA State"=w332:i32, "TDU State"=w329:i32, "PNA Channel"=w326:i32)
            n72 = case shown="True" w338 {
              tunnel: ["FALSE" ("element") "TRUE" ("element")] -> w337
              frame False {
              }
              frame True {
              }
            }
            n73 = Number To Decimal String(number=w348) -> (decimal integer string=w349:string)  [unwired: 1 in]
            n74 = Number To Decimal String(number=w326) -> (decimal integer string=w328:string)  [unwired: 1 in]
            n75 = Number To Decimal String(number=w354) -> (decimal integer string=w355:string)  [unwired: 1 in]
            n76 = Number To Decimal String(number=w347) -> (decimal integer string=w346:string)  [unwired: 1 in]
            n77 = Build Array("TX_DRIVER_AMP_BIAS" ("element"), w349) -> (w322:string[])
            n78 = Number To Decimal String(number=w342) -> (decimal integer string=w341:string)  [unwired: 1 in]
            n79 = Build Array("PNA_CHANNEL" ("element"), w328) -> (w314:string[])
            n80 = Number To Decimal String(number=w329) -> (decimal integer string=w331:string)  [unwired: 1 in]
            n81 = Number To Decimal String(number=w359) -> (decimal integer string=w358:string)  [unwired: 1 in]
            n82 = Build Array("RX_OUTPUT_AMP_BIAS" ("element"), w355) -> (w324:string[])
            n83 = Number To Decimal String(number=w351) -> (decimal integer string=w352:string)  [unwired: 1 in]
            n84 = Build Array("RX_LNA_BIAS" ("element"), w346) -> (w321:string[])
            n85 = Number To Decimal String(number=w332) -> (decimal integer string=w333:string)  [unwired: 1 in]
            n86 = Build Array("TDU_STATE" ("element"), w331) -> (w315:string[])
            n87 = Build Array("MODE" ("element"), w343) -> (w320:string[])
            n88 = Build Array("VGA_STATE" ("element"), w341) -> (w319:string[])
            n89 = Build Array("RX_LNA_BIAS" ("element"), w358) -> (w325:string[])
            n90 = Build Array("TX_INPUT_PA_BIAS" ("element"), w352) -> (w323:string[])
            n91 = Build Array("DSA_STATE" ("element"), w333) -> (w316:string[])
            n92 = Build Array("SWEPT_TOGETHER" ("element"), w337) -> (w318:string[])
            n93 = Build Array("RF_PATH" ("element"), w335) -> (w317:string[])
            n94 = Build Array(w325, w324, w323, w322, w321, w320, w319, w318, w317, w316, w315, w314) -> (w306:string[][])
            n95 = Strip Path(path=w297) -> (name=w284:string)  [unwired: 1 out]
            n96 = String Length(string=w284) -> (length=w287:i32)
            n97 = Subtract(x=w287, y=10) -> (x-y=w285:i32)
            n98 = String Subset(string=w284, length (rest)=w285) -> (substring=w283:string)  [unwired: 1 in]
            n99 = Concatenate Strings(w283, "_DUT_parameters.csv" ("string")) -> (w303:string)
            n100 = Concatenate Strings(w283, "_scantimestamp.csv" ("string")) -> (w299:string)
            n101 = Build Path(base path=w297, name or relative path=w303) -> (appended path=w302:path)
            n102 = Build Path(base path=w297, name or relative path=w299) -> (appended path=w292:path)
            n103 = call-poly <vilib>:"Write Delimited Spreadsheet.vi"("file path (dialog if empty)"=w292, "format (%s)"="%s" ("format (%.3f)"), "1D data"=w289, "append to file? (new file:F)"=FALSE, "error in (no error)"=w291, "transpose? (no:F)"=FALSE, "delimiter (\\t)"="," ("delimiter (\\t)")) -> ("error out"=w290:errorcluster)  [unwired: 7 in, 1 out]
            n104 = call-poly <vilib>:"Write Delimited Spreadsheet.vi"("file path (dialog if empty)"=w302, "format (%s)"="%s" ("format (%.3f)"), "2D data"=w306, "append to file? (new file:F)"=FALSE, "error in (no error)"=w290, "transpose? (no:F)"=FALSE, "delimiter (\\t)"="," ("delimiter (\\t)")) -> ("error out"=w305:errorcluster)  [unwired: 7 in, 1 out]
          }
        }
        n105 = local read "EndRecord"() -> (w26:bool)
      }
      n106 = call "Digital - Cleanup.vi"("Error In"=w19, "Instrument Handle In"=w22) -> ()  [unwired: 10 in]
    }
    frame Enabled {
    }
  }
  n107 = while {
    shift-right: [w375] -> w4
    shift-left: w7 -> [w369]
    shift-right: [w374] -> w17
    shift-left: T2 [] ("VISAPowerInfoInputArray") -> [w376]
    shift-right: [w371] -> _
    shift-left: "Standby" -> [w372]
    shift-right: [w368] -> _
    shift-left: path "" ("appended path") -> [w367]
    shift-right: [w365] -> _
    shift-left: string[][] [] ("Parameter Configuration Echo") -> [w363]
    shift-right: [w366] -> _
    shift-left: "" ("Configuration Echo") -> [w364]
    stop <- "End Program" stop-if-true
    n108 = case shown="\"AttemptRecord\"" w372 {
      tunnel: w376 -> [w399 w407 w429 w496 w672]
      tunnel: w369 -> [w398 w403 w431 w497 w668]
      tunnel: [w397 w404 w430 w495 w623] -> w375
      tunnel: [w396 w407 w429 w496 w672] -> w374
      tunnel: "Record Data Toggle" -> [_ w406 _ w494 _]
      tunnel: ["Standby" w405 w432 w493 "Standby"] -> w371
      tunnel: [path "" ("new file path (Not A Path if cancelled)") path "" ("new file path (Not A Path if cancelled)") w422 w490 w665] -> w368
      tunnel: w367 -> [_ _ w421 w491 w665]
      tunnel: [w378 w401 w420 w489 "" ("Configuration Echo")] -> w366
      tunnel: [w377 w400 w419 w488 string[][] [] ("Parameter Configuration Echo")] -> w365
      tunnel: w364 -> [_ w401 w420 w489 w631]
      tunnel: w363 -> [_ w400 w419 w488 w638]
      frame "Configure" {
        n109 = Build Array("Current Limit Channel 1 (A)", "Current Limit Channel 2 (A)", "Current Limit Channel 3 (A)") -> (w393:dbl[])
        n110 = Build Array("Voltage Channel 1 (V)", "Voltage Channel 2 (V)", "Voltage Channel 3 (V)") -> (w392:dbl[])
        n111 = Build Array(w392, w393) -> (w394:dbl[][])
        n112 = Transpose 2D Array(2D array=w394) -> (transposed array=w391:dbl[][])
        n113 = call "VISA_Keithley2230G_ConfigureInstrument_V1.vi"("VISA resource name"="VISA resource name", "VISAPowerInfoInputArray"=w399, "Input Array (Voltage,Current_Limit)"=w391, "Combination Scheme"="Combination Scheme", "Which Channels to Parallelize"="Which Channels to Parallelize", "error in"=w398, "POWER STATUS IN"="POWER STATUS IN") -> ("POWER STATUS OUT"=→"POWER STATUS OUT":bool, "VISAPowerInfoOutputArray"=w396:T2, "Configuration Echo"=w378:string, "Parameter Configuration Echo"=w377:string[][], "error out"=w397:errorcluster)  [unwired: 8 in]
        "Parameter Configuration Echo" <- w377
        "Configuration Echo" <- w378
      }
      frame "Standby", Default {
        (unwired) cluster{timestamp[], string[]}[] [] ("array")
        n114 = case shown="False" "Apply Power Settings" {
          tunnel: w406 -> [w412 _]
          tunnel: [w411 "Configure"] -> w405
          tunnel: [w410 w417] -> w404
          tunnel: w403 -> [w409 w417]
          frame False {
            n115 = case shown="True" w412 {
              tunnel: ["Standby" "AttemptRecord"] -> w411
              tunnel: [w413 w415] -> w410
              tunnel: w409 -> [w413 w415]
              frame False {
              }
              frame True {
              }
            }
          }
          frame True {
          }
        }
      }
      frame "AttemptRecord" {
        n116 = Array Size(array=w429) -> (size(s)=w433:i32)
        n117 = Two Button Dialog(message="Please check the filepath and the run number. Are these accurate? ", 1:"No" ("F button name (\"Cancel\")"), 2:"Yes" ("T button name (\"OK\")")) -> (T button?=w424:bool)
        n118 = Not Equal To 0?(x=w433) -> (x != 0?=w425:bool)
        n119 = And(x=w425, y=w424) -> (x .and. y?=w423:bool)
        n120 = case shown="True" w423 {
          tunnel: ["Standby" w454] -> w432
          tunnel: w431 -> [w439 w449]
          tunnel: [w436 w460] -> w430
          tunnel: [w435 w458] -> w422
          tunnel: w421 -> [w435 _]
          frame False {
            n121 = call "Display Message to User"("error in (no error)"=w439, "Message"="Initialize/Configure the Keithley Power Supply") -> ("error out"=w437:errorcluster)  [unwired: 8 in, 1 out]
            n122 = property on="Record Data Toggle" class="Bool (strict)"(error in=w437, "Value"=FALSE ("Record Data Toggle")) -> (error out=w436:errorcluster)  [unwired: 1 in, 1 out]
          }
          frame True {
            n123 = Number To Decimal String(number="Run Number") -> (decimal integer string=w443:string)  [unwired: 1 in]
            n124 = Concatenate Strings("Run_" ("Run Number"), w443) -> (w441:string)
            n125 = Concatenate Strings(w441, "_powersupplydata.csv" ("string")) -> (w451:string)
            n126 = List Folder(path="Head FilePath", error in=w449) -> (path out=w447:path, folder names=w445:string[], error out=w448:errorcluster)  [unwired: 2 in, 1 out]
            n127 = Build Path(base path=w447, name or relative path=w441) -> (appended path=w446:path)
            "RunPath" <- w446
            n128 = for {
              shift-right: [w485] -> w456
              shift-left: w448 -> [w485]
              shift-right: [w484] -> w455
              shift-left: w446 -> [w484]
              tunnel: w445 -> [w482] mode=indexing
              tunnel: w441 -> [w483]
              shift-right: [w480] -> w452
              shift-left: FALSE -> [w479]
              n129 = Equal?(x=w482, y=w483) -> (x = y?=w481:bool)
              n130 = case shown="True" w481 {
                selector: w481 -> [_ w487]
                tunnel: [w486 w487] -> w480
                tunnel: w479 -> [w486 _]
                frame False {
                }
                frame True {
                }
              }
            }
            n131 = case shown="False" w452 {
              tunnel: [w471 w474] -> w460
              tunnel: string[] ["Time (H.M.S.###)", "Channel 1 Current (A)", "Channel 1 Voltage (V)", "Channel 2 Current (A)", "Channel 2 Voltage (V)", "Channel 3 Current (A)", "Channel 3 Voltage (V)"] -> [w469 _]
              tunnel: [w467 w477] -> w458
              tunnel: w456 -> [w464 w476]
              tunnel: w455 -> [w463 w477]
              tunnel: ["Record" "Standby"] -> w454
              tunnel: w451 -> [w461 _]
              frame False {
                n132 = Create Folder(path (use dialog)=w463, error in=w464) -> (created path=w466:path, error out=w472:errorcluster)  [unwired: 1 in, 1 out]
                n133 = Build Path(base path=w466, name or relative path=w461) -> (appended path=w465:path)
                n134 = call-poly <vilib>:"Write Delimited Spreadsheet.vi"("file path (dialog if empty)"=w465, "format (%s)"="%s" ("format (%.3f)"), "1D data"=w469, "error in (no error)"=w472, "delimiter (\\t)"="," ("delimiter (\\t)")) -> ("new file path (Not A Path if cancelled)"=w467:path, "error out"=w471:errorcluster)  [unwired: 9 in]
              }
              frame True {
                n135 = call "Display Message to User2"("error in (no error)"=w476) -> ("error out"=w475:errorcluster)  [unwired: 9 in, 1 out]
                n136 = property on="Record Data Toggle" class="Bool (strict)"(error in=w475, "Value"=FALSE ("Record Data Toggle")) -> (error out=w474:errorcluster)  [unwired: 1 in, 1 out]
              }
            }
          }
        }
      }
      frame "Record" {
        n137 = for {
          tunnel: w496 -> [w511] mode=indexing
          shift-right: [w506] -> w492
          shift-left: w497 -> [w509]
          tunnel: w491 -> [w505]
          tunnel: [w504] -> w490
          n138 = Unbundle(w511) -> ("VISA resource name"=w510:refnum<visa-resource-name>)  [unwired: 6 out]
          n139 = flat-sequence {
            tunnel: w509 -> [w513]
            tunnel: [w513] -> w508
            tunnel: [w512] -> w507
            tunnel: w510 -> [w541]
            tunnel: w508 -> [w540]
            tunnel: w507 -> [w530]
            tunnel: w505 -> [w525]
            tunnel: [w526] -> w503
            tunnel: [w524] -> w502
            tunnel: [w565] -> w504
            tunnel: [w562] -> w506
            tunnel: w503 -> [w563]
            tunnel: w502 -> [w565]
            frame #0 {
              n140 = Get Date/Time In Seconds() -> (seconds since 1Jan1904=w512:timestamp)
            }
            frame #1 {
              w514 = 0.01 ("Delay Time (s)")
              n141 = VISA Write(VISA resource name=w541, write buffer="FETCH:CURR? ALL", error in (no error)=w540) -> (VISA resource name out=w544:refnum<visa-resource-name>, error out=w543:errorcluster)  [unwired: 1 out]
              n142 = VISA Read(VISA resource name=w544, byte count=u32 100, error in (no error)=w543) -> (VISA resource name out=w535:refnum<visa-resource-name>, read buffer=w520:string, error out=w532:errorcluster)  [unwired: 1 out]
              n143 = disable-structure shown="Enabled" {
                disable-tunnel: w532 -> [w547 w548]
                disable-tunnel: [w546 w548] -> w531
                disable-tunnel: w514 -> [w545 _]
                frame Enabled {
                  n144 = call "Time Delay"("error in (no error)"=w547, "Delay Time (s)"=w545) -> ("error out"=w546:errorcluster)  [unwired: 9 in]
                }
                frame Disabled {
                }
              }
              n145 = VISA Write(VISA resource name=w535, write buffer="FETCH:VOLT? ALL", error in (no error)=w531) -> (VISA resource name out=w537:refnum<visa-resource-name>, error out=w538:errorcluster)  [unwired: 1 out]
              n146 = String Length(string=w520) -> (length=w522:i32)
              n147 = Decrement(x=w522) -> (x-1=w521:i32)
              n148 = VISA Read(VISA resource name=w537, byte count=u32 100, error in (no error)=w538) -> (read buffer=w517:string, error out=w533:errorcluster)  [unwired: 2 out]
              n149 = String Subset(string=w520, length (rest)=w521) -> (substring=w516:string)  [unwired: 1 in]
              n150 = String Length(string=w517) -> (length=w519:i32)
              n151 = Decrement(x=w519) -> (x-1=w518:i32)
              n152 = String Subset(string=w517, length (rest)=w518) -> (substring=w515:string)  [unwired: 1 in]
              n153 = Format Date/Time String(time format string (%c)="%H.%M.%S%8u", seconds (now)=w530) -> (date/time string=w529:string)  [unwired: 1 in]
              n154 = disable-structure shown="Enabled" {
                disable-tunnel: w533 -> [w551 w552]
                disable-tunnel: w514 -> [w550 _]
                disable-tunnel: [w549 w552] -> w527
                frame Enabled {
                  n155 = call "Time Delay2"("error in (no error)"=w551, "Delay Time (s)"=w550) -> ("error out"=w549:errorcluster)  [unwired: 9 in]
                }
                frame Disabled {
                }
              }
              n156 = Build Array(w529, w516, w515) -> (w523:string[])
              "appended array" <- w523
              n157 = disable-structure shown="Enabled" {
                disable-tunnel: [w560 w561] -> w526
                disable-tunnel: w527 -> [w559 w561]
                disable-tunnel: w525 -> [w557 _]
                disable-tunnel: [w555 _] -> w524
                disable-tunnel: w523 -> [w554 _]
                frame Enabled {
                  n158 = call-poly <vilib>:"Write Delimited Spreadsheet.vi"("file path (dialog if empty)"=w557, "format (%s)"="%s" ("format (%.3f)"), "1D data"=w554, "append to file? (new file:F)"=TRUE, "error in (no error)"=w559, "delimiter (\\t)"="," ("delimiter (\\t)")) -> ("new file path (Not A Path if cancelled)"=w555:path, "error out"=w560:errorcluster)  [unwired: 8 in]
                }
                frame Disabled {
                }
              }
            }
            frame #2 {
              n159 = case shown="True" "BeamStart" {
                tunnel: w565 -> [_ w611]
                tunnel: [w590 w600] -> w564
                tunnel: w563 -> [w590 w604]
                frame False {
                }
                frame True {
                  n160 = Strip Path(path=w611) -> (stripped path=w610:path, name=w591:string)
                  n161 = Get Date/Time In Seconds() -> (seconds since 1Jan1904=w609:timestamp)
                  n162 = String Length(string=w591) -> (length=w597:i32)
                  n163 = Subtract(x=w597, y=20) -> (x-y=w595:i32)
                  n164 = String Subset(string=w591, length (rest)=w595) -> (substring=w594:string)  [unwired: 1 in]
                  n165 = Concatenate Strings(w594, "_timestart.txt" ("name or relative path")) -> (w592:string)
                  n166 = Build Path(base path=w610, name or relative path=w592) -> (appended path=w603:path)
                  n167 = Format Date/Time String(time format string (%c)="%H.%M.%S%8u", seconds (now)=w609) -> (date/time string=w598:string)  [unwired: 1 in]
                  n168 = Open/Create/Replace File(file path (use dialog)=w603, error in=w604, operation (0:open)=T6."open or create", access (0:read/write)=enum16{"read/write", "read-only", "write-only"}."read/write") -> (refnum out=w599:refnum<file>, error out=w605:errorcluster)  [unwired: 2 in, 1 out]
                  n169 = Write to Text File(file (use dialog)=w599, text=w598, error in=w605) -> (refnum out=w606:refnum<file>, error out=w607:errorcluster)  [unwired: 1 in, 1 out]
                  n170 = Close File(refnum=w606, error in=w607) -> (error out=w600:errorcluster)  [unwired: 1 out]
                }
              }
              n171 = case shown="True" "BeamEnd" {
                tunnel: w565 -> [_ w589]
                tunnel: w564 -> [w568 w582]
                tunnel: [w568 w580] -> w562
                frame False {
                }
                frame True {
                  n172 = Strip Path(path=w589) -> (stripped path=w588:path, name=w571:string)
                  n173 = String Length(string=w571) -> (length=w572:i32)
                  n174 = Get Date/Time In Seconds() -> (seconds since 1Jan1904=w585:timestamp)
                  n175 = Subtract(x=w572, y=20) -> (x-y=w574:i32)
                  n176 = String Subset(string=w571, length (rest)=w574) -> (substring=w573:string)  [unwired: 1 in]
                  n177 = Concatenate Strings(w573, "_timeend.txt" ("name or relative path")) -> (w569:string)
                  n178 = Build Path(base path=w588, name or relative path=w569) -> (appended path=w586:path)
                  n179 = Format Date/Time String(time format string (%c)="%H.%M.%S%8u", seconds (now)=w585) -> (date/time string=w583:string)  [unwired: 1 in]
                  n180 = Open/Create/Replace File(file path (use dialog)=w586, error in=w582, operation (0:open)=T6."open or create", access (0:read/write)=enum16{"read/write", "read-only", "write-only"}."read/write") -> (refnum out=w587:refnum<file>, error out=w581:errorcluster)  [unwired: 2 in, 1 out]
                  n181 = Write to Text File(file (use dialog)=w587, text=w583, error in=w581) -> (refnum out=w579:refnum<file>, error out=w578:errorcluster)  [unwired: 1 in, 1 out]
                  n182 = Close File(refnum=w579, error in=w578) -> (error out=w580:errorcluster)  [unwired: 1 out]
                }
              }
            }
          }
        }
        n183 = case shown="False" w494 {
          tunnel: [w499 w501] -> w495
          tunnel: w492 -> [w499 w501]
          tunnel: ["PostProcess" "Record"] -> w493
          frame False {
          }
          frame True {
          }
        }
      }
      frame "PostProcess" {
        n184 = call-poly <vilib>:"Read Delimited Spreadsheet.vi"("file path (dialog if empty)"=w665, "format (%s)"="%s", "number of rows (all:-1)"=-1, "error in (no error)"=w668) -> ("all rows"=w655:string[][], "error out"=w667:errorcluster)  [unwired: 6 in, 4 out]
        n185 = Index Array(array=w655, index (col)=0 ("index (row)")) -> (element=w654:string[])  [unwired: 1 in]
        n186 = Delete From Array(array=w654, index=0) -> (array with subset deleted=w652:string[])  [unwired: 1 in, 1 out]
        n187 = for {
          shift-right: [w691] -> w657
          shift-left: w667 -> [w690]
          shift-right: [w692] -> _
          shift-left: 0.0 -> [w693]
          tunnel: w652 -> [w687] mode=indexing
          tunnel: [w680] -> w649 mode=indexing
          i -> [w706]
          n188 = Search/Split String(string=w687, search string/char (-)=",") -> (substring before match=w684:string, match + rest of string=w681:string)  [unwired: 1 in, 1 out]
          n189 = Equal To 0?(x=w706) -> (x = 0?=w705:bool)
          n190 = Search/Split String(string=w684, search string/char (-)=".") -> (substring before match=w709:string, match + rest of string=w708:string, offset of match=w712:i32)  [unwired: 1 in]
          n191 = Increment(x=w712) -> (x+1=w711:i32)
          n192 = Decimal String To Number(string=w709, offset=0) -> (number=w702:i32)  [unwired: 1 in, 1 out]
          n193 = Search/Split String(string=w708, search string/char (-)=".", offset (0)=w711) -> (substring before match=w707:string, match + rest of string=w703:string)  [unwired: 1 out]
          n194 = Multiply(x=60, y=w702) -> (x*y=w697:i32)
          n195 = Decimal String To Number(string=w707, offset=0) -> (number=w701:i32)  [unwired: 1 in, 1 out]
          n196 = Fract/Exp String To Number(string=w703, offset=1) -> (number=w695:dbl)  [unwired: 2 in, 1 out]
          n197 = Multiply(x=60, y=w701) -> (x*y=w698:i32)
          n198 = Add(x=w697, y=w698) -> (x+y=w696:i32)
          n199 = Add(x=w696, y=w695) -> (x+y=w694:dbl)
          n200 = case shown="True" w705 {
            tunnel: w694 -> [w715 w720]
            tunnel: w693 -> [w716 w718]
            tunnel: [w716 w720] -> w692
            tunnel: [w717 w719] -> w691
            tunnel: w690 -> [w717 w719]
            tunnel: [w714 w718] -> w685
            frame False {
              n201 = Subtract(x=w715, y=w716) -> (x-y=w714:dbl)
            }
            frame True {
            }
          }
          n202 = Number To Fractional String(number=w685) -> (F-format string=w682:string)  [unwired: 3 in]
          n203 = Concatenate Strings(w684, "," ("string"), w682, w681, "\r\n") -> (w680:string)
        }
        n204 = Concatenate Strings("Time (H.M.S.###),Elapsed Time (s),Channel 1 Current (A),Channel 1 Voltage (V),Channel 2 Current (A),Channel 2 Voltage (V),Channel 3 Current (A),Channel 3 Voltage (V)" ("new element/subarray"), "\r\n") -> (w646:string)
        n205 = Insert Into Array(array=w649, index=0, new element=w646) -> (w648:string[])
        n206 = Strip Path(path=w665) -> (stripped path=w615:path, name=w661:string)
        n207 = String Length(string=w661) -> (length=w664:i32)
        n208 = Subtract(x=w664, y=4) -> (x-y=w662:i32)
        n209 = String Subset(string=w661, length (rest)=w662) -> (substring=w624:string)  [unwired: 1 in]
        n210 = Concatenate Strings(w624, "_augment.csv" ("string")) -> (w659:string)
        n211 = Build Path(base path=w615, name or relative path=w659) -> (appended path=w658:path)
        n212 = Concatenate Strings(w624, "_parameters.csv" ("name or relative path")) -> (w639:string)
        n213 = Strip Path(path=w615) -> (name=w612:string)  [unwired: 1 out]
        n214 = Concatenate Strings(w624, "_channel_config.txt" ("name or relative path")) -> (w626:string)
        n215 = Build Path(base path=w615, name or relative path=w639) -> (appended path=w643:path)
        n216 = Build Path(base path=w615, name or relative path=w626) -> (appended path=w630:path)
        n217 = call-poly <vilib>:"Write Delimited Spreadsheet.vi"("file path (dialog if empty)"=w658, "1D data"=w648, "error in (no error)"=w657, "delimiter (\\t)"="," ("delimiter (\\t)")) -> ("error out"=w632:errorcluster)  [unwired: 10 in, 1 out]
        n218 = Concatenate Strings(w612, "_CopyFolder" ("name or relative path")) -> (w613:string)
        n219 = Open/Create/Replace File(file path (use dialog)=w630, error in=w632, operation (0:open)=T6."open or create", access (0:read/write)=enum16{"read/write", "read-only", "write-only"}."read/write") -> (refnum out=w633:refnum<file>, error out=w634:errorcluster)  [unwired: 2 in, 1 out]
        n220 = Write to Text File(file (use dialog)=w633, text=w631, error in=w634) -> (refnum out=w635:refnum<file>, error out=w636:errorcluster)  [unwired: 1 in, 1 out]
        n221 = Close File(refnum=w635, error in=w636) -> (error out=w637:errorcluster)  [unwired: 1 out]
        n222 = Build Path(base path=w615, name or relative path=w613) -> (appended path=w622:path)
        n223 = call-poly <vilib>:"Write Delimited Spreadsheet.vi"("file path (dialog if empty)"=w643, "format (%s)"="%s", "2D data"=w638, "error in (no error)"=w637, "delimiter (\\t)"="," ("delimiter (\\t)")) -> ("error out"=w619:errorcluster)  [unwired: 9 in, 1 out]
        n224 = List Folder(path=w615, error in=w619) -> (path out=w618:path, filenames=w616:string[], error out=w617:errorcluster)  [unwired: 2 in, 1 out]
        n225 = Create Folder(path (use dialog)=w622, error in=w617) -> (created path=w620:path, error out=w621:errorcluster)  [unwired: 1 in, 1 out]
        n226 = for {
          tunnel: w620 -> [w676]
          tunnel: w618 -> [w675]
          shift-right: [w678] -> w623
          shift-left: w621 -> [w677]
          tunnel: w616 -> [w673] mode=indexing
          n227 = Build Path(base path=w675, name or relative path=w673) -> (appended path=w674:path)
          n228 = Copy(8:w677, 10:w676, 11:w674) -> (0:w678:errorcluster)  [unwired: 2 in, 2 out]
        }
      }
    }
    "Status" <- w371
    "VISAPowerInfoInputArray" <- w374
    "EndRecord" <- "End Program"
  }
  n229 = Merge Errors(w4, w2) -> (w3:errorcluster)
  n230 = for {
    tunnel: w17 -> [w727] mode=indexing
    shift-right: [w721] -> w15
    shift-left: w3 -> [w722]
    n231 = Unbundle(w727) -> ("VISA resource name"=w725:refnum<visa-resource-name>)  [unwired: 6 out]
    n232 = VISA Write(VISA resource name=w725, write buffer="OUTP OFF", error in (no error)=w722) -> (VISA resource name out=w724:refnum<visa-resource-name>, error out=w723:errorcluster)  [unwired: 1 out]
    n233 = VISA Close(VISA resource name=w724, error in (no error)=w723) -> (error out=w721:errorcluster)
  }
  n234 = call <vilib>:"Simple Error Handler.vi"("error in (no error)"=w15) -> ()  [unwired: 4 in, 5 out]
